vi "CleanUp.vi"(0 "class data in":refnum<class "Game.lvclass">, 5 "error in":errorcluster) -> (14 "class data out":refnum<class "Game.lvclass">, 19 "error out":errorcluster)   [LabVIEW 2010, in "Labricks.lvlib" / "Game.lvclass"]
uses:
  Game.lvclass
  Game.lvclass/Game.ctl
  RenderBase/SceneRoot_class/SceneRoot.lvclass
  RenderBase/SceneObject_class/SceneObject.lvclass
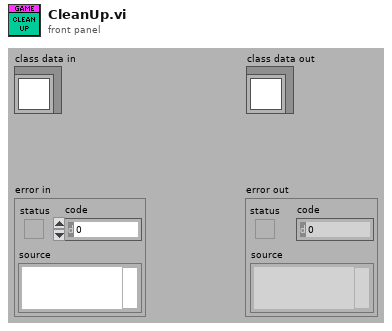
[diagram p1: front panel]
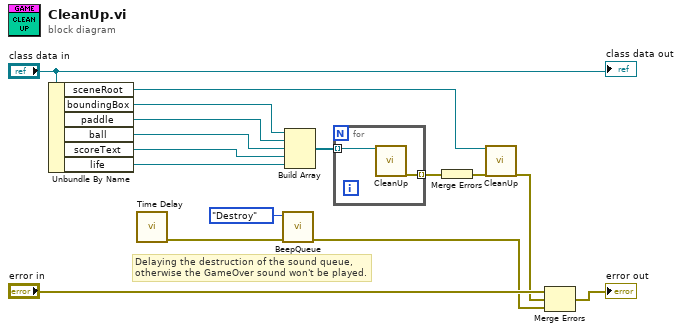
[diagram p0: block diagram]
diagram:
  # "Delaying the destruction of the sound queue,\notherwise the GameOver sound won't be played."
  n1 = Unbundle By Name("class data in") -> ("sceneRoot"=w4:refnum<class "SceneRoot.lvclass">, "boundingBox"=w11:refnum<class "BoundingBox.lvclass">, "paddle"=w10:refnum<class "Paddle.lvclass">, "ball"=w9:refnum<class "Ball.lvclass">, "scoreText"=w8:refnum<class "Text.lvclass">, "life"=w7:refnum<class "Text.lvclass">)
  n2 = call "Time Delay"() -> ("error out"=w13:errorcluster)  [unwired: 11 in]
  n3 = call "BeepQueue.vi"("error in"=w13, "mode in (Get)"=enum16{"Get", "Init", "Destroy"}."Destroy") -> ("error out"=w2:errorcluster)  [unwired: 4 in, 1 out]
  n4 = Build Array(w11, w10, w9, w8, w7) -> (w6:refnum<class "SceneObject.lvclass">[])
  n5 = for {
    tunnel: w6 -> [w18] mode=indexing
    tunnel: [w17] -> w5 mode=indexing
    n6 = call-dynamic "CleanUp.vi"("class data in"=w18) -> ("error out"=w17:errorcluster)  [unwired: 17 in, 1 out]
  }
  n7 = Merge Errors(w5) -> (w1:errorcluster)
  n8 = call-dynamic "CleanUp.vi"("class data in"=w4, "error in"=w1) -> ("error out"=w3:errorcluster)  [unwired: 16 in, 1 out]
  n9 = Merge Errors("error in", w3, w2) -> (→"error out":errorcluster)
  "class data out" <- "class data in"
